vi "Write Calibration.vi"(4 "DSPic Measurements":dbl[](array[numeric]), 5 "String Cal Mode":string, 6 "Actual Measurements":dbl[](array[numeric]), 7 "Position in":u32, 8 "error in (no error)":errorcluster, 9 "Calibration Type":string, 10 "Cree Comms in":refnum<class "Cree Communications.lvclass">, 11 "Calibration in":refnum<class "Calibration.lvclass">) -> (0 "error out":errorcluster)   [LabVIEW 2015, in "Calibration.lvclass"]
uses:
  Calibration.lvclass
  Classes/Cree Communications/Class/Cree Communications.lvclass
  Classes/Cree Communications/Cree Comms Messages/Set Vsec Offset/Set Vsec Offset.lvclass
  Classes/Cree Communications/Cree Comms Messages/Set Vsec Scalar/Set Vsec Scalar.lvclass
  Classes/Cree Communications/Cree Comms Messages/CC Message/CC Message.lvclass/CC Message.ctl
  Classes/Cree Communications/Cree Comms Messages/Set String Current Scalar/Set String Current Scalar.lvclass
  Classes/Cree Communications/Cree Comms Messages/Set String Current Offset/Set String Current Offset.lvclass
  Classes/Cree Communications/Cree Comms Messages/Set ITemp Scalar/Set ITemp Scalar.lvclass
  Classes/Cree Communications/Cree Comms Messages/Set ITemp Offset/Set ITemp Offset.lvclass
  Classes/Cree Communications/Cree Comms Messages/CC Message/CC Message.lvclass
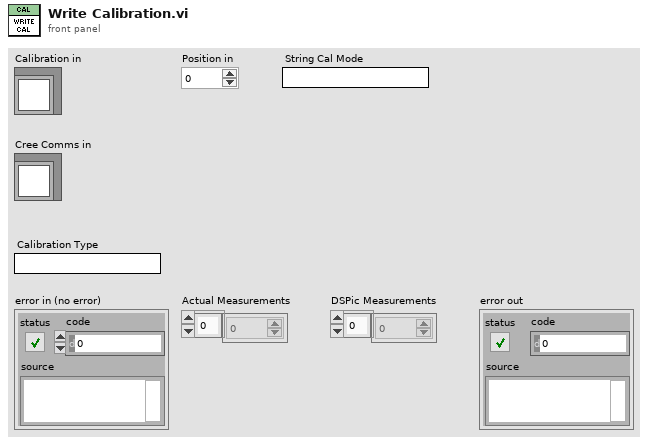
[diagram p1: front panel]
types:
  T1 = cluster{"Offset":dbl, "String":enum16{"Red", "BSY1", "BSY2"}}
  T2 = cluster{"Scalar":dbl, "String":enum16{"Red", "BSY1", "BSY2"}}
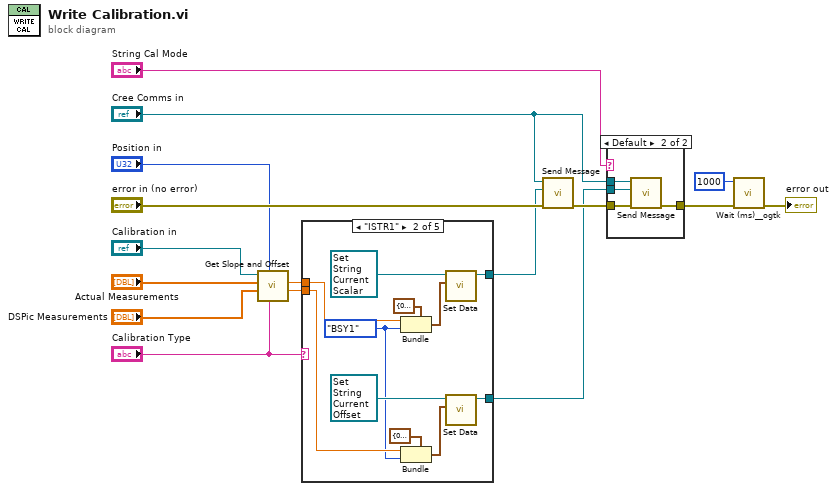
[diagram p0: block diagram]
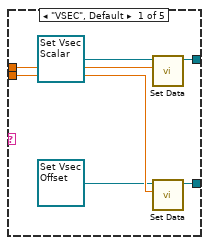
[diagram p3: hidden frame]
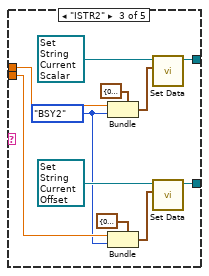
[diagram p4: hidden frame]
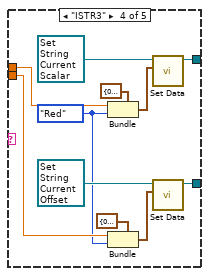
[diagram p5: hidden frame]
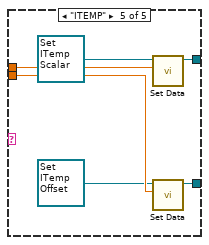
[diagram p6: hidden frame]
diagram:
  n1 = call "Get Slope and Offset.vi"("Calibration Type"="Calibration Type", "Position"="Position in", "DSpic Measurements"="DSPic Measurements", "Measurements"="Actual Measurements", "Calibration in"="Calibration in") -> ("Offset"=w8:dbl, "Scalar"=w9:dbl)  [unwired: 3 in, 2 out]
  n2 = case shown="\"ISTR1\"" "Calibration Type" {
    tunnel: [w22 w31 w42 w53 w61] -> w7
    tunnel: [w21 w30 w41 w52 w60] -> w6
    tunnel: w9 -> [w20 w32 w43 w54 w59]
    tunnel: w8 -> [w19 w25 w36 w47 w58]
    frame "VSEC", Default {
      n3 = call "Set Data.vi"("Data"=w20, "CC Message in"=refnum<class "Set Vsec Scalar.lvclass"> refnum ("Cree Comms Messages.lvlib:Set Vsec Scalar.lvclass")) -> ("CC Message out"=w22:refnum<class "Set Vsec Scalar.lvclass">)  [unwired: 8 in, 1 out]
      n4 = call "Set Data.vi"("Data"=w19, "CC Message in"=refnum<class "Set Vsec Offset.lvclass"> refnum ("Cree Comms Messages.lvlib:Set Vsec Offset.lvclass")) -> ("CC Message out"=w21:refnum<class "Set Vsec Offset.lvclass">)  [unwired: 8 in, 1 out]
    }
    frame "ISTR1" {
      w23 = enum16{"Red", "BSY1", "BSY2"}."BSY1" ("String")
      n5 = Bundle(cluster=T2 {"Scalar"=0.0, "String"=enum."Red"} ("Message Type"), "Scalar"=w32, "String"=w23) -> (w27:T2)
      n6 = Bundle(cluster=T1 {"Offset"=0.0, "String"=enum."Red"} ("Message Type"), "Offset"=w25, "String"=w23) -> (w24:T1)
      n7 = call "Set Data.vi"("Data"=w27, "CC Message in"=refnum<class "Set String Current Scalar.lvclass"> refnum ("Cree Comms Messages.lvlib:Set String Current Scalar.lvclass")) -> ("CC Message out"=w31:refnum<class "Set String Current Scalar.lvclass">)  [unwired: 8 in, 1 out]
      n8 = call "Set Data.vi"("Data"=w24, "CC Message in"=refnum<class "Set String Current Offset.lvclass"> refnum ("Cree Comms Messages.lvlib:Set String Current Offset.lvclass")) -> ("CC Message out"=w30:refnum<class "Set String Current Offset.lvclass">)  [unwired: 8 in, 1 out]
    }
    frame "ISTR2" {
      w34 = enum16{"Red", "BSY1", "BSY2"}."BSY2" ("String")
      n9 = Bundle(cluster=T2 {"Scalar"=0.0, "String"=enum."Red"} ("Message Type"), "Scalar"=w43, "String"=w34) -> (w38:T2)
      n10 = Bundle(cluster=T1 {"Offset"=0.0, "String"=enum."Red"} ("Message Type"), "Offset"=w36, "String"=w34) -> (w35:T1)
      n11 = call "Set Data.vi"("Data"=w38, "CC Message in"=refnum<class "Set String Current Scalar.lvclass"> refnum ("Cree Comms Messages.lvlib:Set String Current Scalar.lvclass")) -> ("CC Message out"=w42:refnum<class "Set String Current Scalar.lvclass">)  [unwired: 8 in, 1 out]
      n12 = call "Set Data.vi"("Data"=w35, "CC Message in"=refnum<class "Set String Current Offset.lvclass"> refnum ("Cree Comms Messages.lvlib:Set String Current Offset.lvclass")) -> ("CC Message out"=w41:refnum<class "Set String Current Offset.lvclass">)  [unwired: 8 in, 1 out]
    }
    frame "ISTR3" {
      w45 = enum16{"Red", "BSY1", "BSY2"}."Red" ("String")
      n13 = Bundle(cluster=T2 {"Scalar"=0.0, "String"=enum."Red"} ("Message Type"), "Scalar"=w54, "String"=w45) -> (w49:T2)
      n14 = Bundle(cluster=T1 {"Offset"=0.0, "String"=enum."Red"} ("Message Type"), "Offset"=w47, "String"=w45) -> (w46:T1)
      n15 = call "Set Data.vi"("Data"=w49, "CC Message in"=refnum<class "Set String Current Scalar.lvclass"> refnum ("Cree Comms Messages.lvlib:Set String Current Scalar.lvclass")) -> ("CC Message out"=w53:refnum<class "Set String Current Scalar.lvclass">)  [unwired: 8 in, 1 out]
      n16 = call "Set Data.vi"("Data"=w46, "CC Message in"=refnum<class "Set String Current Offset.lvclass"> refnum ("Cree Comms Messages.lvlib:Set String Current Offset.lvclass")) -> ("CC Message out"=w52:refnum<class "Set String Current Offset.lvclass">)  [unwired: 8 in, 1 out]
    }
    frame "ITEMP" {
      n17 = call "Set Data.vi"("Data"=w59, "CC Message in"=refnum<class "Set ITemp Scalar.lvclass"> refnum ("Cree Comms Messages.lvlib:Set ITemp Scalar.lvclass")) -> ("CC Message out"=w61:refnum<class "Set ITemp Scalar.lvclass">)  [unwired: 8 in, 1 out]
      n18 = call "Set Data.vi"("Data"=w58, "CC Message in"=refnum<class "Set ITemp Offset.lvclass"> refnum ("Cree Comms Messages.lvlib:Set ITemp Offset.lvclass")) -> ("CC Message out"=w60:refnum<class "Set ITemp Offset.lvclass">)  [unwired: 8 in, 1 out]
    }
  }
  n19 = call "Send Message.vi"("error in (no error)"="error in (no error)", "Cree Comms Message"=w7, "Acrobat Template in"="Cree Comms in") -> ("error out"=w13:errorcluster)  [unwired: 7 in, 1 out]
  n20 = case shown="Default" "String Cal Mode" {
    tunnel: "Cree Comms in" -> [_ w66]
    tunnel: w13 -> [w62 w65]
    tunnel: w6 -> [_ w64]
    tunnel: [w62 w63] -> w5
    frame "SinglePoint" {
    }
    frame Default {
      n21 = call "Send Message.vi"("error in (no error)"=w65, "Cree Comms Message"=w64, "Acrobat Template in"=w66) -> ("error out"=w63:errorcluster)  [unwired: 7 in, 1 out]
    }
  }
  n22 = call <userlib>:"Wait (ms)__ogtk.vi"("error in (no error)"=w5, "milliseconds to wait"=u32 1000) -> ("error out"=→"error out":errorcluster)  [unwired: 8 in, 1 out]
